vi "Set SG Path.vi"(0 "Path in":refnum<class "SA 18GHz Path.lvclass">, 5 "Cal point in":T1, 11 "error in":errorcluster) -> (4 "Path out":refnum<class "SA 18GHz Path.lvclass">, 6 "Cal point out":T1, 8 "Source Gain":dbl, 10 "Digital Gain":dbl, 15 "error out":errorcluster)   [LabVIEW 2023, in "RFFixtureCharact.RFPM.lvlib" / "SA 18GHz Path.lvclass"]
uses:
  SA 18GHz Path.lvclass
  Public/Base Classes/Scalar/Scalar Path/Type Definitions/Cal Point.ctl
  C:/srd-semi-rfcal-software/AuxTools/STSRFFixtureCharactUtility/Source/Code Modules/Common/Base Classes/Path/Path.lvclass
  C:/srd-semi-rfcal-software/AuxTools/STSRFFixtureCharactUtility/Source/Code Modules/Fixture/Public/Base Classes/Scalar/SA Abstract Path/SA Abstract Path.lvclass
  Charact Result Accessor/Base/Charact Result Accessor.lvclass
  Public/Base Classes/Scalar/SA Abstract Path/SA Abstract Path.lvclass/SA Abstract Path.ctl
  Public/Base Classes/Scalar/SA Abstract Path/Properties/Read Cal Tone Pin.vi
  <instrlib>/niRFPM/niRFPM.llb/NI-RFPM Set TX Path By Switch Path String.vi
  Common/Result Accessor/Result Accessor.lvclass
  Public/Base Classes/Scalar/Scalar Path/Scalar Path.lvclass
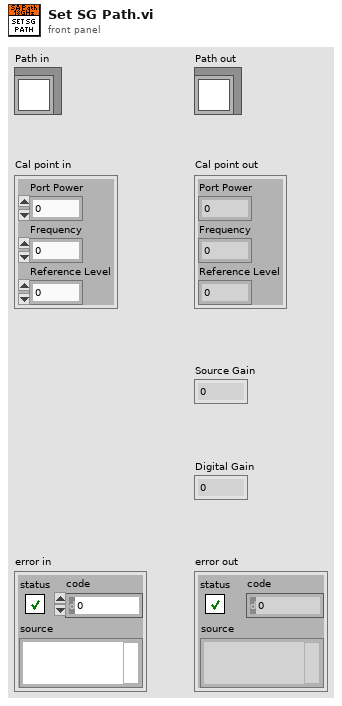
[diagram p1: front panel]
types:
  T1 = typedef "RFFixtureCharact.Public.lvlib/Scalar Path.lvclass/Cal Point.ctl" = cluster{"Port Power":dbl, "Frequency":dbl, "Reference Level":dbl}
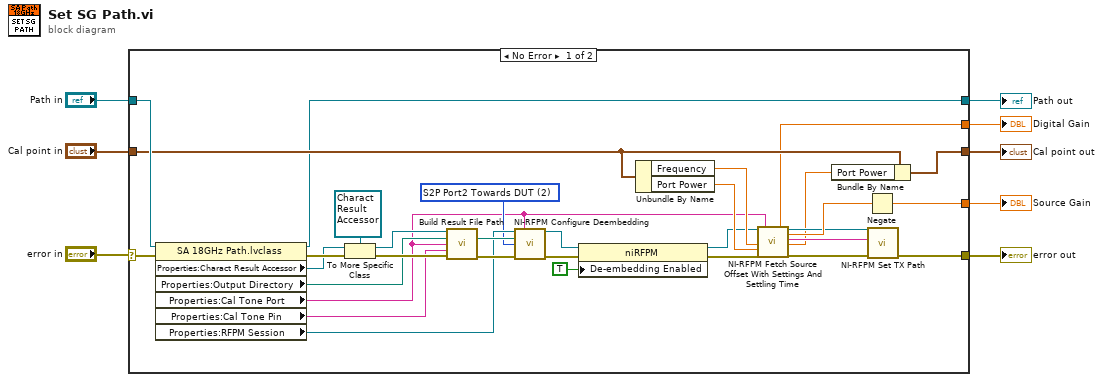
[diagram p0: block diagram]
diagram:
  n1 = case shown="No Error" "error in" {
    selector: "error in" -> [w32 w43]
    tunnel: [w33 w43] -> w2
    tunnel: [w22 w42] -> w4
    tunnel: "Path in" -> [w31 w42]
    tunnel: [w34 _] -> w3
    tunnel: "Cal point in" -> [w30 w41]
    tunnel: [w28 w41] -> w1
    tunnel: [w27 _] -> w5
    frame No Error {
      w10 = 2 items=["S2P Port1 Towards DUT"=1, "S2P Port2 Towards DUT"=2] ("Deembedding Orientation")
      n2 = property class="SA 18GHz Path.lvclass"(reference=w31, error in=w32) -> (reference out=w22:refnum<class "SA 18GHz Path.lvclass">, error out=w23:errorcluster, "Properties:Charact Result Accessor"=w21:refnum<class "Result Accessor.lvclass">, "Properties:Output Directory"=w20:path, "Properties:Cal Tone Port"=w9:string, "Properties:Cal Tone Pin"=w19:string, "Properties:RFPM Session"=w16:refnum<k15>)
      n3 = To More Specific Class(target class=refnum<class "Charact Result Accessor.lvclass"> refnum ("Charact Result Accessor in"), reference=w21, error in=w23) -> (specific class reference=w25:refnum<class "Charact Result Accessor.lvclass">, error out=w24:errorcluster)
      n4 = call-dynamic "Build Result File Path.vi"("Charact Result Accessor in"=w25, "Output Directory"=w20, "Port 1"=w9, "Port 2"=w19, "error in (no error)"=w24) -> ("Result File Path"=w17:path, "error out"=w18:errorcluster)  [unwired: 8 in, 1 out]
      n5 = call <instrlib>:"NI-RFPM Configure Deembedding.vi"("instrument handle"=w16, "port"=w9, "Deembedding S2P File Path"=w17, "Deembedding Orientation"=w10, "error in (no error)"=w18) -> ("instrument handle out"=w12:refnum<k15>, "error out"=w15:errorcluster)  [unwired: 9 in]
      n6 = property class="niRFPM"(reference=w12, error in=w15, "De-embedding Enabled"=TRUE ("Measurement:De-embedding Enabled")) -> (reference out=w13:refnum<k15>, error out=w14:errorcluster)
      n7 = Unbundle By Name(w30) -> ("Frequency"=w40:dbl, "Port Power"=w39:dbl)
      n8 = call <instrlib>:"NI-RFPM Fetch Source Offset With Settings And Settling Time.vi"("instrument handle"=w13, "Frequency"=w40, "Power"=w39, "error in"=w14, "Port"=w9) -> ("Digital Gain"=w27:dbl, "instrument handle out"=w35:refnum<k15>, "Source Offset"=w38:dbl, "Switch Path String"=w37:string, "Calibrated Power"=w29:dbl, "error out"=w36:errorcluster)  [unwired: 8 in, 1 out]
      n9 = Bundle By Name(cluster=w30, "Port Power"=w29) -> (w28:T1)
      n10 = Negate(x=w38) -> (-x=w34:dbl)
      n11 = call-poly <instrlib>:"NI-RFPM Set TX Path.vi"("instrument handle"=w35, "TX Switch Path"=w37, "error in (no error)"=w36) -> ("error out"=w33:errorcluster)  [unwired: 11 in, 1 out]
    }
    frame Error {
    }
  }
  "error out" <- w2
  "Source Gain" <- w3
  "Cal point out" <- w1
  "Digital Gain" <- w5
  "Path out" <- w4
